vi "Create.vi"(8 "error in (no error)":errorcluster, 11 "Model Directory":path=path "") -> (0 "error out":errorcluster, 3 "New QR Code Detector":refnum<class "QR Code Detector.lvclass">)   [LabVIEW 2020, in "g_ar_toolkit.feature_detection.lvlib" / "QR Code Detector.lvclass"]
uses:
  QR Code Detector.lvclass
  QR Code Detector.lvclass/QR Code Detector.ctl
  g_ar_toolkit.common/g_ar_toolkit.common.lvlib
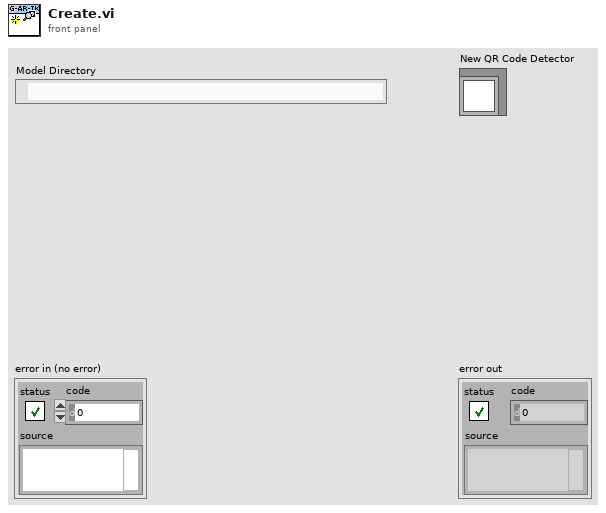
[diagram p1: front panel]
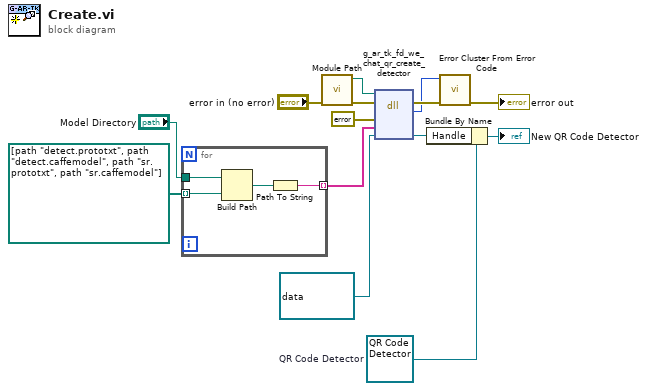
[diagram p0: block diagram]
diagram:
  w14 = refnum<class "QR Code Detector.lvclass"> refnum  # QR Code Detector
  n1 = for {
    tunnel: "Model Directory" -> [w18]
    tunnel: [w16] -> w2 mode=indexing
    tunnel: path[] [path "detect.prototxt", path "detect.caffemodel", path "sr.prototxt", path "sr.caffemodel"] -> [w15] mode=indexing
    n2 = Build Path(base path=w18, name or relative path=w15) -> (appended path=w17:path)
    n3 = Path To String(path=w17) -> (string=w16:string)
  }
  n4 = call "Module Path.vi"("error in (no error)"="error in (no error)") -> ("error out"=w5:errorcluster, "Path"=w4:path)  [unwired: 9 in]
  n5 = dll-call lib="?" fn="g_ar_tk_fd_we_chat_qr_create_detector" ("g_ar_toolkit.*.*:g_ar_tk_capture_context_create")(path in=w4, error in=w5, "error_cluster"=errorcluster {"status"=FALSE, "code"=0, "source"=""} ("error constant"), "paths"=w2, "EDVR"=refnum<data-value> refnum) -> (error out=w11:errorcluster, "MgErr"=w7:i32, "EDVR"=w9:refnum<data-value>)  [unwired: 3 in, 1 out]
  n6 = Bundle By Name(cluster=w14, "Handle"=w9) -> (→"New QR Code Detector":refnum<class "QR Code Detector.lvclass">)
  n7 = call <vilib>:"Error Cluster From Error Code.vi"("error in (no error)"=w11, "error code (0)"=w7) -> ("error out"=→"error out":errorcluster)  [unwired: 7 in]
